vi "Z6_Beamline.color Southtower BL.vi"(0 "i ref in":refnum<vi>, 2 "Color State Southtower Input":i32, 5 "error in (no error)":errorcluster) -> (14 "i ref out":refnum<vi>, 16 "Color State Southwower Exit":i32, 19 "error out":errorcluster)   [LabVIEW 2014, in "Z6_Beamline.lvlib"]
doc: "This Vi colors the Mirrortower beamline elements."
uses:
  Z6_Beamline.lvlib
  PH_StatusHandler/PH_StatusHandler.Status.ctl
  PH_Common/PH_Common.lvlib
  PH_StatusHandler/PH_StatusHandler.lvlib
  PH_BL-Master/PH_BL-Master.lvlib
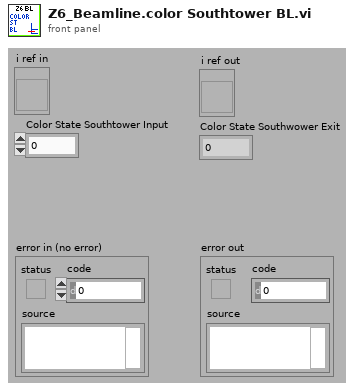
[diagram p1: front panel]
types:
  T1 = typedef "PH_StatusHandler.lvlib/PH_StatusHandler.Status.ctl" = i16
  T2 = typedef "Z6_Beamline.lvlib/Z6_Beamline.i attribute.ctl" = cluster{"Subs ok GUI Refs":T3, "Refs BL Northtower":refnum<vi>[], "Refs BL Southtower":refnum<vi>[], "Refs BL 100TW COS":refnum<vi>[], "State Subsystems":cluster{"Northtower":bool, "Southtower":bool, "Frontends":bool, "100TW COS":bool}, "Z6 Beamline Status Subscriber Information":T4, "Color State PHELIX":i16}
  T3 = typedef "Z6_Beamline.lvlib/Z6_Beamline.Subsystem ok GUI Refs.ctl" = cluster{"Northtower ok":refnum<vi>, "Southtower ok":refnum<vi>, "Frontends ok":refnum<vi>, "100TW COS ok":refnum<vi>}
  T4 = typedef "Z6_Beamline.lvlib/Z6_Beamline.Status Subscriber Information.ctl" = cluster{"BL Z6 Shutter":T5, "CH 10":T5, "CH 11":T5, "ST Flip Cam":T5, "ST Flip DB":T5, "BL Z6 Dump":T5}
  T5 = typedef "PH_BL-Master.lvlib/PH_BL-Master.Status Subscriber Information.ctl" = cluster{"Index of element":i32, "Attributeset":T6}
  T6 = typedef "PH_BL-Master.lvlib/PH_BL-Master.Attribute Set.ctl" = enum16{"Boolean Status Service Subscriber", "Picture Status Service Subscriber"}
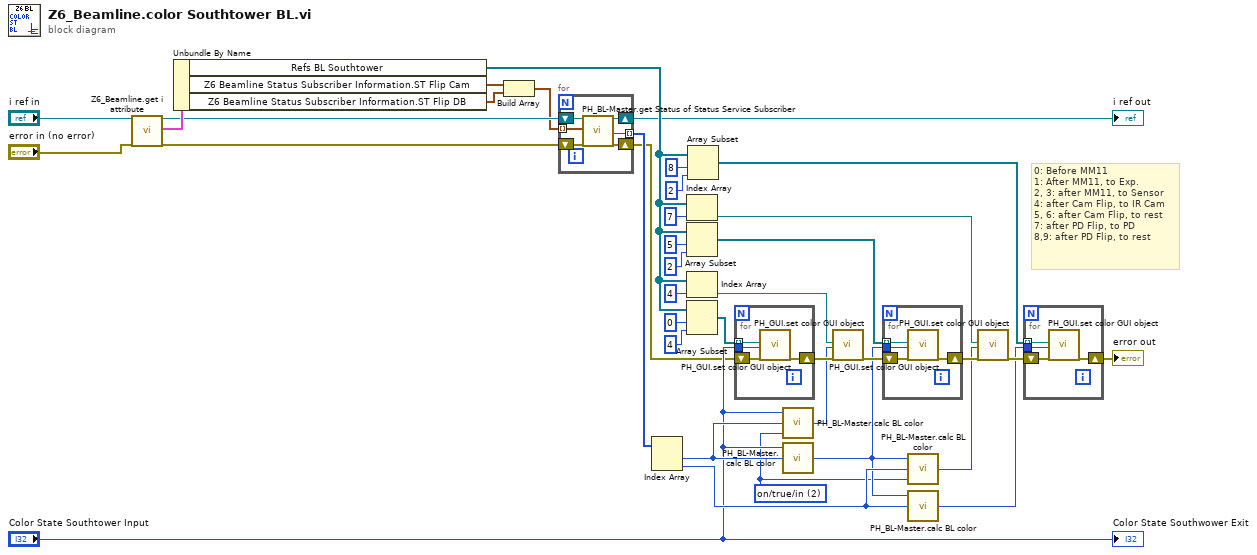
[diagram p0: block diagram]
diagram:
  w10 = T1 2 items=["no info", "off/false/out", "on/true/in", "Failure", "Alarm", "Status 1", "Status 2", "Status 3"] ("State ABLE")
  # "0: Before MM11\n1: After MM11, to Exp.\n2, 3: after MM11, to Sensor\n4: after Cam Flip, to IR Cam\n5, 6: after Cam Flip, to rest\n7: after PD Flip, to PD\n8,9: after PD Flip, to rest"
  n1 = call "Z6_Beamline.get i attribute.vi"("i ref in"="i ref in", "error in (no error)"="error in (no error)") -> ("i ref out"=w7:refnum<vi>, "i attribute"=w38:T2, "error out"=w6:errorcluster)  [unwired: 15 in]
  n2 = Unbundle By Name(w38) -> ("Refs BL Southtower"=w19:refnum<vi>[], "Z6 Beamline Status Subscriber Information.ST Flip Cam"=w3:T5, "Z6 Beamline Status Subscriber Information.ST Flip DB"=w2:T5)
  n3 = Build Array(w3, w2) -> (w1:T5[])
  n4 = for {
    shift-right: [w43] -> w4
    shift-left: w6 -> [w44]
    shift-right: [w41] -> w5
    shift-left: w7 -> [w42]
    tunnel: w1 -> [w40] mode=indexing
    tunnel: [w39] -> w28 mode=indexing
    n5 = call "PH_BL-Master.get Status of Status Service Subscriber.vi"("i ref in"=w42, "Wanted Status Subscriber Information"=w40, "error in (no error)"=w44) -> ("i ref out"=w41:refnum<vi>, "Status"=w39:T1, "error out"=w43:errorcluster)  [unwired: 11 in, 3 out]
  }
  "i ref out" <- w5
  n6 = Index Array(array=w28) -> (element #1=w24:T1, element #2=w23:T1)  [unwired: 2 in]
  n7 = Index Array(array=w19, index=7) -> (element=w14:refnum<vi>)
  n8 = Array Subset(array=w19, index=5, length=2) -> (w25:refnum<vi>[])
  n9 = Index Array(array=w19, index=4) -> (element=w26:refnum<vi>)
  n10 = Array Subset(array=w19, index=0, length=4) -> (w31:refnum<vi>[])
  n11 = Array Subset(array=w19, index=8, length=2) -> (w12:refnum<vi>[])
  n12 = for {
    tunnel: w31 -> [w48] mode=indexing
    shift-right: [w46] -> w30
    shift-left: w4 -> [w47]
    tunnel: "Color State Southtower Input" -> [w45]
    n13 = call "PH_GUI.set color GUI object.vi"("GUI object Ref"=w48, "State"=w45, "error in (no error)"=w47) -> ("error out"=w46:errorcluster)  [unwired: 16 in]
  }
  n14 = call "PH_BL-Master.calc BL color.vi"("State for \"2\" (on) of ABLE (off/false/out)"=w10, "State ABLE"=w24, "State before ABLE"="Color State Southtower Input") -> ("State after ABLE"=w29:i32)
  n15 = call "PH_BL-Master.calc BL color.vi"("State ABLE"=w24, "State before ABLE"="Color State Southtower Input") -> ("State after ABLE"=w22:i32)  [unwired: 1 in]
  n16 = call "PH_GUI.set color GUI object.vi"("GUI object Ref"=w26, "State"=w29, "error in (no error)"=w30) -> ("error out"=w27:errorcluster)  [unwired: 16 in]
  n17 = for {
    tunnel: w25 -> [w52] mode=indexing
    shift-right: [w50] -> w16
    shift-left: w27 -> [w51]
    tunnel: w22 -> [w49]
    n18 = call "PH_GUI.set color GUI object.vi"("GUI object Ref"=w52, "State"=w49, "error in (no error)"=w51) -> ("error out"=w50:errorcluster)  [unwired: 16 in]
  }
  n19 = call "PH_BL-Master.calc BL color.vi"("State for \"2\" (on) of ABLE (off/false/out)"=w10, "State ABLE"=w23, "State before ABLE"=w22) -> ("State after ABLE"=w13:i32)
  n20 = call "PH_BL-Master.calc BL color.vi"("State ABLE"=w23, "State before ABLE"=w22) -> ("State after ABLE"=w11:i32)  [unwired: 1 in]
  n21 = call "PH_GUI.set color GUI object.vi"("GUI object Ref"=w14, "State"=w13, "error in (no error)"=w16) -> ("error out"=w15:errorcluster)  [unwired: 16 in]
  n22 = for {
    tunnel: w12 -> [w56] mode=indexing
    shift-right: [w54] -> w17
    shift-left: w15 -> [w55]
    tunnel: w11 -> [w53]
    n23 = call "PH_GUI.set color GUI object.vi"("GUI object Ref"=w56, "State"=w53, "error in (no error)"=w55) -> ("error out"=w54:errorcluster)  [unwired: 16 in]
  }
  "error out" <- w17
  "Color State Southwower Exit" <- "Color State Southtower Input"
